vi "config_save_state.vi"(6 "appended path":path, 7 "General state cluster":T1 {"Channel" items=["A"=1, "B"=2, "A + B"=3, "C"=4, "A + C"=5, "A + B"=6, "D"=8, "A + D"=9, "B + D"=10, "C + D"=12, "A + B + C + D"=15]; "FFT Down Sample" min=1 max=8 step=1; "window" items=["Rectangle"=0, "Hanning"=1, "Hamming"=2, "Blackman-Harris"=3, "Exact Blackman"=4, "Blackman"=5, "Flat Top"=6, "4 Term B-Harris "=7, "7 Term B-Harris"=8, "Low Sidelobe"=9, "Blackman Nuttall"=11, "Triangle"=30, "Bartlett-Hanning"=31, "Bohman"=32, "Parzen"=33, "Welch"=34, "Kaiser"=60, "Dolph-Chebyshev"=61, "Gaussian"=62]; "Galvo params only for file storage"."n_dataset" min=1; "Galvo params only for file storage"."X center" format="%^_3g"; "Galvo params only for file storage"."X span" format="%^_3g"; "Galvo params only for file storage"."Y center" format="%^_3g"; "Galvo params only for file storage"."Y span" format="%^_3g"; "ATS_clock"."Source" items=["Internal"=1, "Fast External"=2, "Medium External"=3, "Slow External"=4, "External AC"=5, "External DC"=6, "External 10MHz"=7, "Internal 10MHz"=8]; "ATS_clock"."Sample Rate" items=["1 kS/s"=1, "2 kS/s"=2, "5 kS/s"=4, "10 kS/s"=8, "20 kS/s"=10, "50 kS/s"=12, "100 kS/s"=14, "200 kS/s"=16, "500 kS/s"=18, "1 MS/s"=20, "2 MS/s"=24, "5 MS/s"=26, "10 MS/s"=28, "20 MS/s"=30, "50 MS/s"=34, "100 MS/s"=36, "125 MS/s"=37, "200 MS/s"=40, "500 MS/s"=48, "800 MS/s"=50, "1000 MS/s"=53, "1200 MS/s"=55, "1500 MS/s"=58, "2000 MS/s"=63, "2400 MS/s"=106, "3000 MS/s"=117, "3600 MS/s"=123, "4000 MS/s"=128, "USER_DEF"=0]; "ATS_clock"."Edge" items=["Rising", "Falling"]; "ATS_clock"."Rate Ext Ref" items=["0.4G"=400000000, "0.8G"=800000000, "1.2G"=1200000000, "1.6G"=1600000000, "2.0G"=2000000000, "2.4G"=2400000000, "2.8G"=2800000000, "3.2G"=3200000000, "3.6G"=3600000000]; "ATS_clock 2"."Source" items=["Internal"=1, "Fast External"=2, "Medium External"=3, "Slow External"=4, "External AC"=5, "External DC"=6, "External 10MHz"=7, "Internal 10MHz"=8]; "ATS_clock 2"."Sample Rate" items=["1 kS/s"=1, "2 kS/s"=2, "5 kS/s"=4, "10 kS/s"=8, "20 kS/s"=10, "50 kS/s"=12, "100 kS/s"=14, "200 kS/s"=16, "500 kS/s"=18, "1 MS/s"=20, "2 MS/s"=24, "5 MS/s"=26, "10 MS/s"=28, "20 MS/s"=30, "50 MS/s"=34, "100 MS/s"=36, "125 MS/s"=37, "200 MS/s"=40, "500 MS/s"=48, "800 MS/s"=50, "1000 MS/s"=53, "1200 MS/s"=55, "1500 MS/s"=58, "2000 MS/s"=63, "2400 MS/s"=106, "3000 MS/s"=117, "3600 MS/s"=123, "4000 MS/s"=128, "USER_DEF"=0]; "ATS_clock 2"."Edge" items=["Rising", "Falling"]; "ATS_clock 2"."Rate Ext Ref" items=["0.4G"=400000000, "0.8G"=800000000, "1.2G"=1200000000, "1.6G"=1600000000, "2.0G"=2000000000, "2.4G"=2400000000, "2.8G"=2800000000, "3.2G"=3200000000, "3.6G"=3600000000]; "AO.type" items=["DMA"=10054, "Interrupts"=10204, "Programmed I/O"=10264, "USB Bulk"=12590]}, 9 "reference 3":refnum<vi>, 10 "reference in":refnum<vi>, 11 "Cluster in":refnum<vi>) -> ()   [LabVIEW 2024]
uses:
  CTRL/Typedefs/OCT_F_state.ctl
  <vilib>/Analysis/4window.llb/windowTd.ctl
  CTRL/Typedefs/ORS_Galvo_params.ctl
  CTRL/Typedefs/ORS_Per_Ch_params.ctl
  <vilib>/Utility/miscctls.llb/LVCursorListTypeDef.ctl
  <vilib>/Analysis/NI_AALPro.lvlib
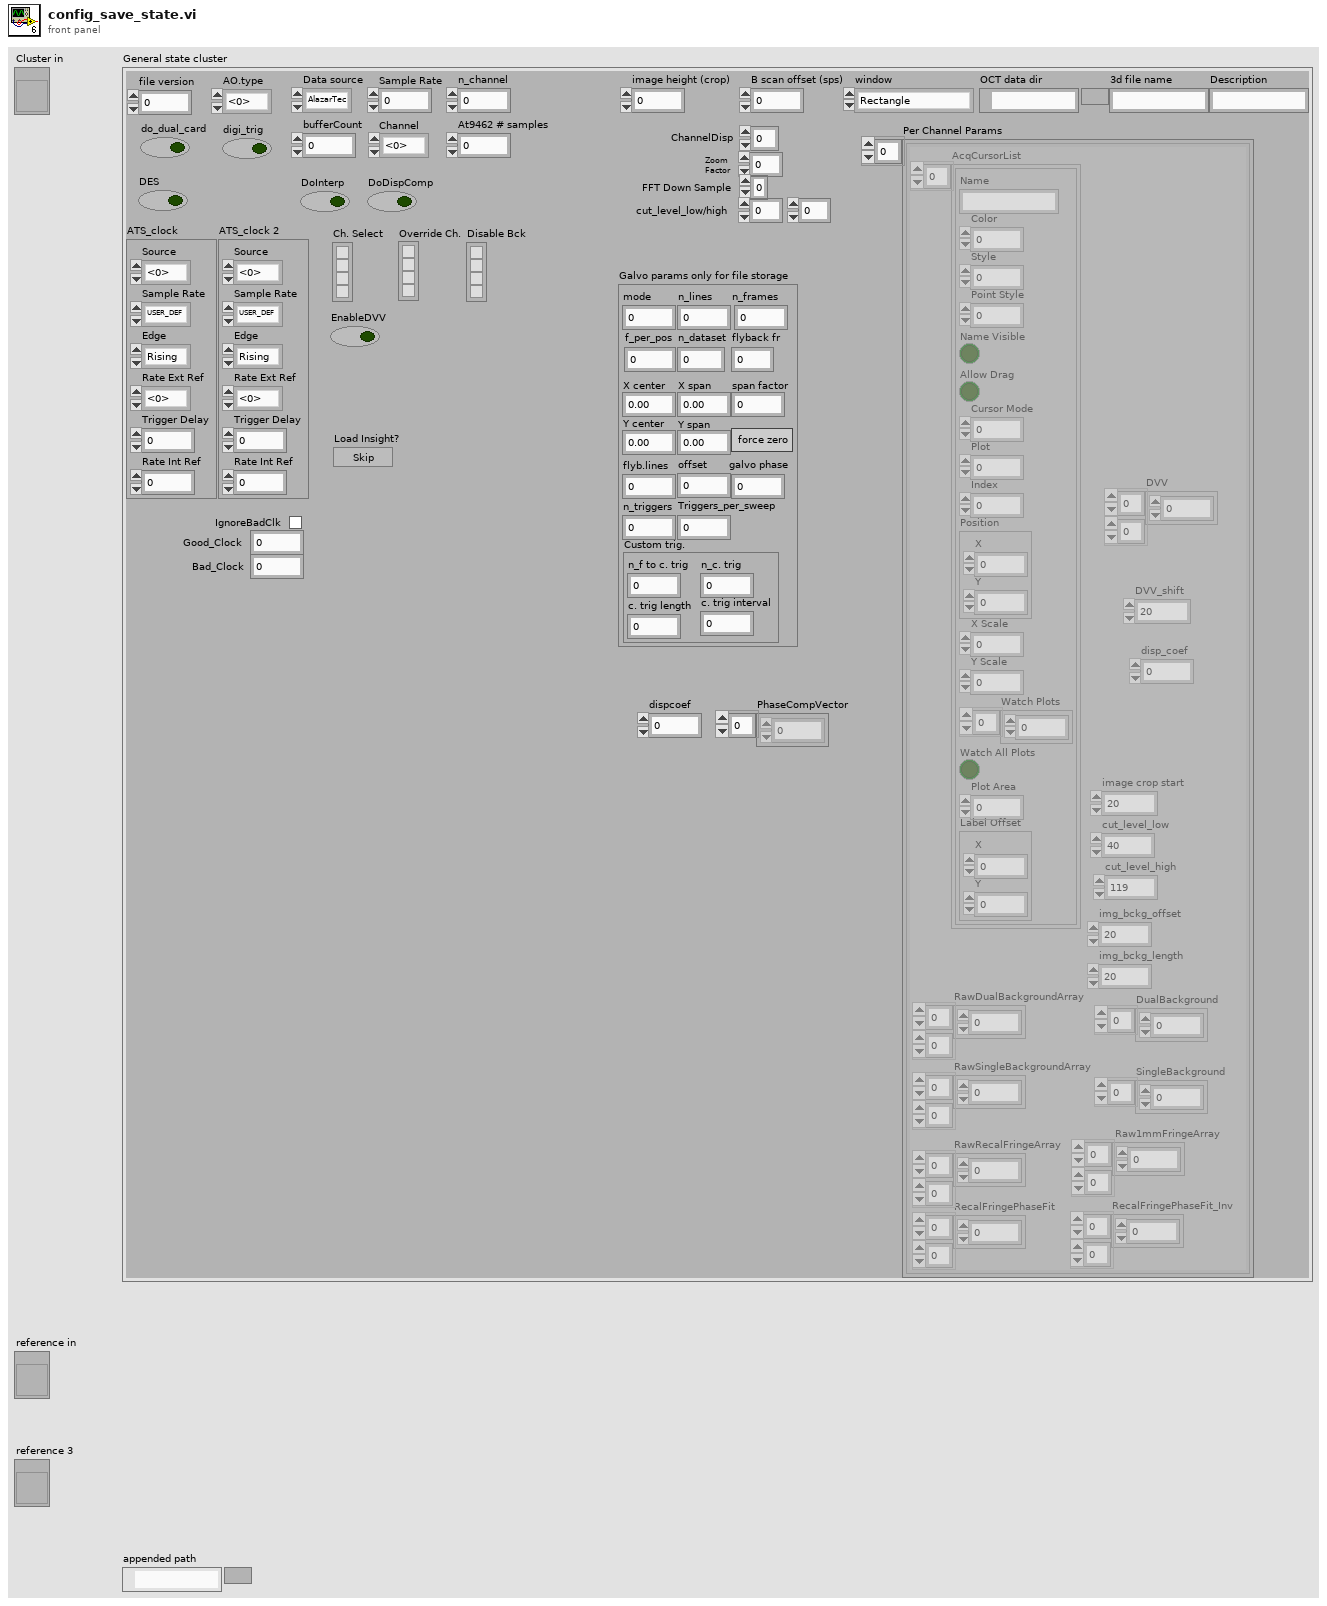
[diagram p1: front panel]
types:
  T1 = typedef "OCT_F_state.ctl" = cluster{"Data source":enum32{"AlazarTec"}, "Sample Rate":dbl, "n_channel":i32, "At9462 # samples":u32, "image height (crop)":i32, "B scan offset (sps)":dbl, "window":T2, "OCT data dir":path, "3d file name":string, "Description":string, "Galvo params only for file storage":T3, "Per Channel Params":T4, "file version":u32, "do_dual_card":bool, "ATS_clock":cluster{"Source":u32, "Sample Rate":u32, "Edge":u32, "Rate Ext Ref":u32, "Trigger Delay":u32, "Rate Int Ref":u32}, "ATS_clock 2":cluster{"Source":u32, "Sample Rate":u32, "Edge":u32, "Rate Ext Ref":u32, "Trigger Delay":u32, "Rate Int Ref":u32}, "DES":bool, "digi_trig":bool, "Ch. Select":bool[], "Override Ch.":bool[], "DoInterp":bool, "EnableDVV":bool, "bufferCount":i32, "dispcoef":dbl, "AO.type":i32, "Disable Bck":bool[], "PhaseCompVector":cdb[], "DoDispComp":bool, "Load Insight?":bool, "ChannelDisp":i32, "Zoom Factor":sgl, "FFT Down Sample":i32, "cut_level_high":dbl, "cut_level_low":dbl, "Channel":u32, "IgnoreBadClk":bool, "Good_Clock":dbl, "Bad_Clock":dbl}
  T2 = typedef "NI_AALPro.lvlib/windowTd.ctl" = u32
  T3 = typedef "ORS_Galvo_params.ctl" = cluster{"n_lines":i32, "n_frames":i32, "force to zero":bool, "Triggers_per_sweep":dbl, "X center":dbl, "X span":dbl, "Y center":dbl, "Y span":dbl, "flyb.lines":i32, "n_triggers":i32, "mode":i32, "offset":dbl, "galvo phase":i32, "span factor":dbl, "Custom trig.":cluster{"n_f to c. trig":i32, "c. trig length":i32, "c. trig interval":i32, "n_c. trig":i32}, "f_per_pos":i32, "n_dataset":u32, "flyback fr":u16}
  T4 = typedef "ORS_Per_Ch_params.ctl" = cluster{"AcqCursorList":T5, "RecalFringePhaseFit_Inv":dbl[][], "RawDualBackgroundArray":i16[][], "RawSingleBackgroundArray":i16[][], "RawRecalFringeArray":i16[][], "RecalFringePhaseFit":dbl[][], "SingleBackground":i16[], "DualBackground":i16[], "image crop start":i32, "cut_level_low":dbl, "cut_level_high":dbl, "Raw1mmFringeArray":i16[][], "img_bckg_offset":i32, "img_bckg_length":i32, "DVV":i16[][], "DVV_shift":i32, "disp_coef":dbl}[]
  T5 = typedef "LVCursorListTypeDef.ctl" = cluster{"Name":string, "Color":u32, "Style":u8, "Point Style":u8, "Name Visible":bool, "Allow Drag":bool, "Cursor Mode":u32, "Plot":i32, "Index":i32, "Position":cluster{"X":dbl, "Y":dbl}, "X Scale":u32, "Y Scale":u32, "Watch Plots":i32[], "Watch All Plots":bool, "Plot Area":i32, "Label Offset":cluster{"X":dbl, "Y":dbl}}[]
  T6 = enum16{"big-endian, network order", "native, host order", "little-endian"}
  T7 = cluster{"AcqCursorList":T5, "RecalFringePhaseFit_Inv":dbl[][], "RawDualBackgroundArray":i16[][], "RawSingleBackgroundArray":i16[][], "RawRecalFringeArray":i16[][], "RecalFringePhaseFit":dbl[][], "SingleBackground":i16[], "DualBackground":i16[], "image crop start":i32, "cut_level_low":dbl, "cut_level_high":dbl, "Raw1mmFringeArray":i16[][], "img_bckg_offset":i32, "img_bckg_length":i32, "DVV":i16[][], "DVV_shift":i32, "disp_coef":dbl}
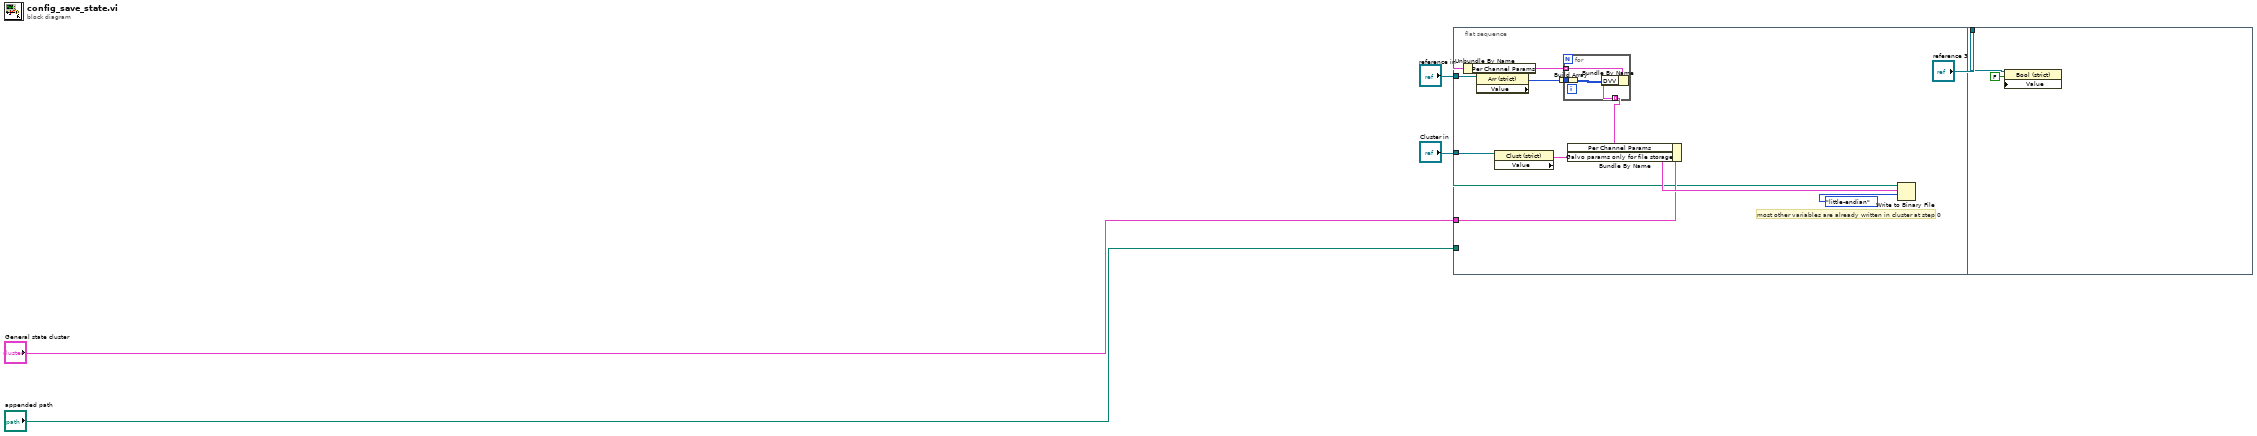
[diagram p0: block diagram]
diagram:
  n1 = flat-sequence {
    tunnel: "General state cluster" -> [w13]
    tunnel: "appended path" -> [w8]
    tunnel: "Cluster in" -> [w7]
    tunnel: "reference in" -> [w6]
    tunnel: "reference 3" -> [w20]
    frame #0 {
      # "most other variables are already written in cluster at step 0"
      n2 = Unbundle By Name(w13) -> ("Per Channel Params"=w12:T4)
      n3 = property class="Arr (strict)"(reference=w6) -> ("Value"=w10:u32[])  [unwired: 1 in, 2 out]
      n4 = property class="Clust (strict)"(reference=w7) -> ("Value"=w14:T3)  [unwired: 1 in, 2 out]
      n5 = Build Array(w10) -> (w9:u32[][])
      n6 = for {
        tunnel: w12 -> [w19] mode=indexing
        tunnel: [w18] -> w11 mode=indexing
        tunnel: w9 -> [w17]
        n7 = Bundle By Name(cluster=w19, "DVV"=w17) -> (w18:T7)
      }
      n8 = Bundle By Name(cluster=w13, "Per Channel Params"=w11, "Galvo params only for file storage"=w14) -> (w15:T1)
      n9 = Write to Binary File(file (use dialog)=w8, data=w15, 9:T6."little-endian" ("byte order (0:big-endian, network order)")) -> ()  [unwired: 3 in, 3 out]
    }
    frame #1 {
      n10 = property class="Bool (strict)"(reference=w20, "Value"=FALSE ("Save state file")) -> ()  [unwired: 1 in, 2 out]
    }
  }
